vi "Lab_3_START_Clusters_Files_SUBVI_Michal_Cedro.vi"(8 "Error IN":errorcluster, 11 "HR Data Structure IN":T1 {"Raw Data"."Time" format="%<%x %.3X>T"}) -> (0 "error out":errorcluster, 3 "HR Data Structure OUT":T1 {"Raw Data"."Time" format="%<%x %.3X>T"})   [LabVIEW 2025]
uses:
  Labview-master/Lab_3/HR_Data_Structure.ctl
  Labview-master/Lab_3/Raw_Data_IN_HR.ctl
  Labview-master/Lab_3/Runner_Data_Structure.ctl
panel:
  out "HEART RATE ZONE":string[][](array[string])
  out "XY Graph":cluster{dbl[], "Heart Rate Zone":i32[]}(graph)
  out "BPM":cluster{"Time":timestamp[], "Bpm":i32[]}(graph)
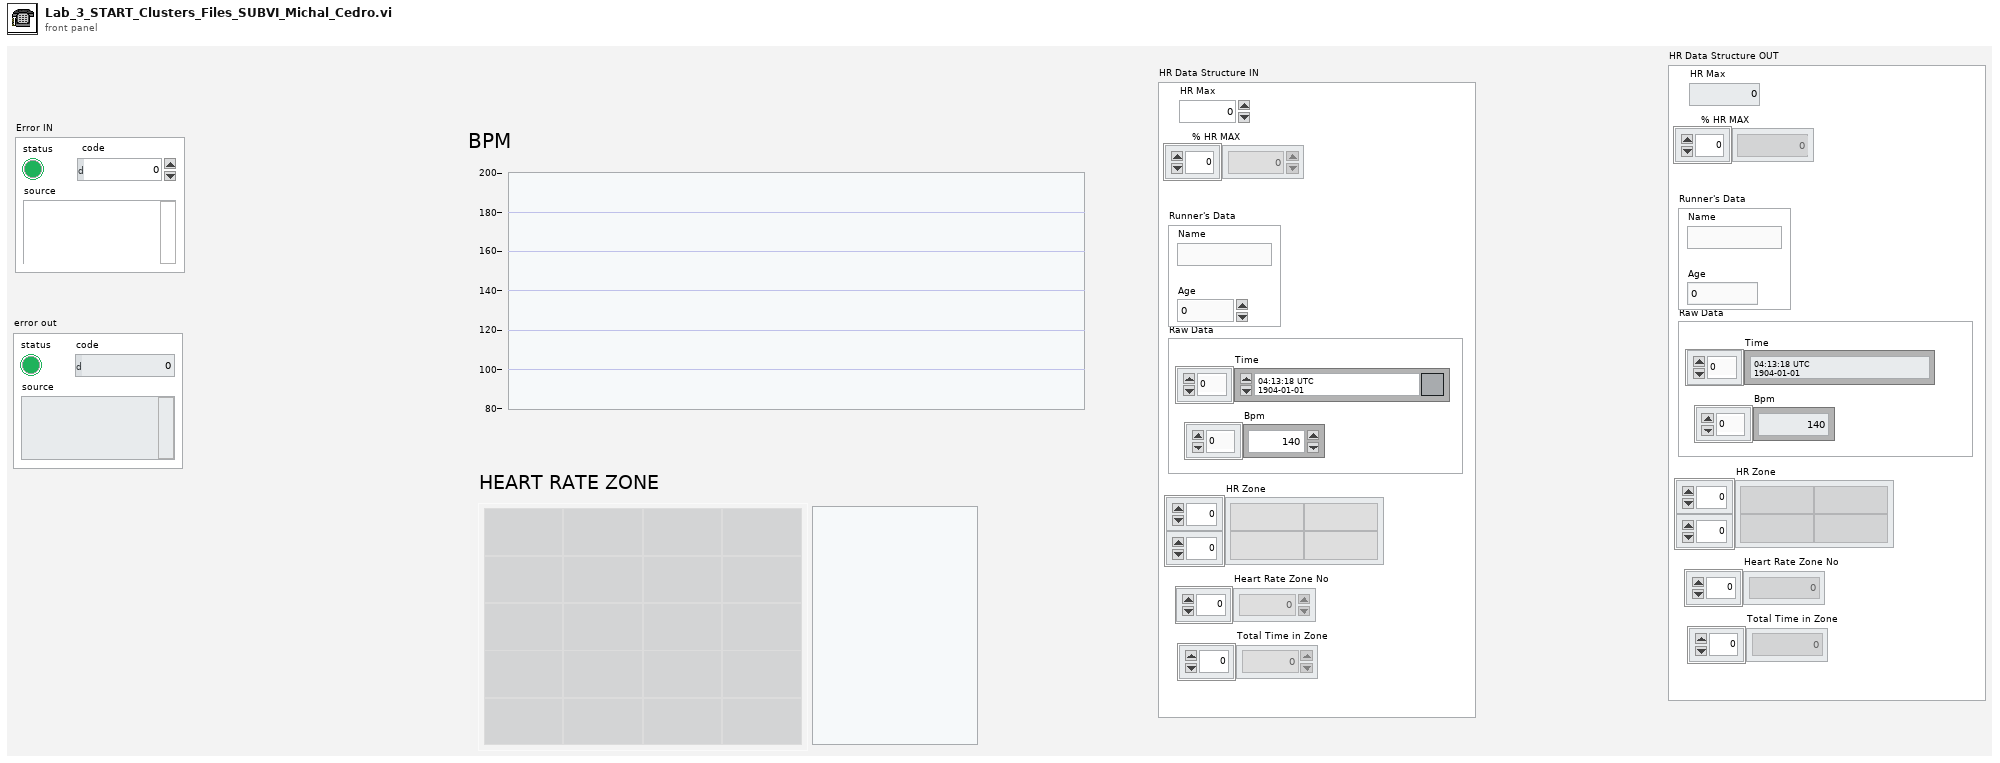
[diagram p1: front panel]
types:
  T1 = typedef "HR_Data_Structure.ctl" = cluster{"HR Max":i32, "% HR MAX ":dbl[], "Raw Data":T2, "Runner's Data":T3, "HR Zone":string[][], "Total Time in Zone":dbl[], "Heart Rate Zone No":dbl[]}
  T2 = typedef "Raw_Data_IN_HR.ctl" = cluster{"Time":timestamp[], "Bpm":i32[]}
  T3 = typedef "Runner_Data_Structure.ctl" = cluster{"Name":string, "Age":i32}
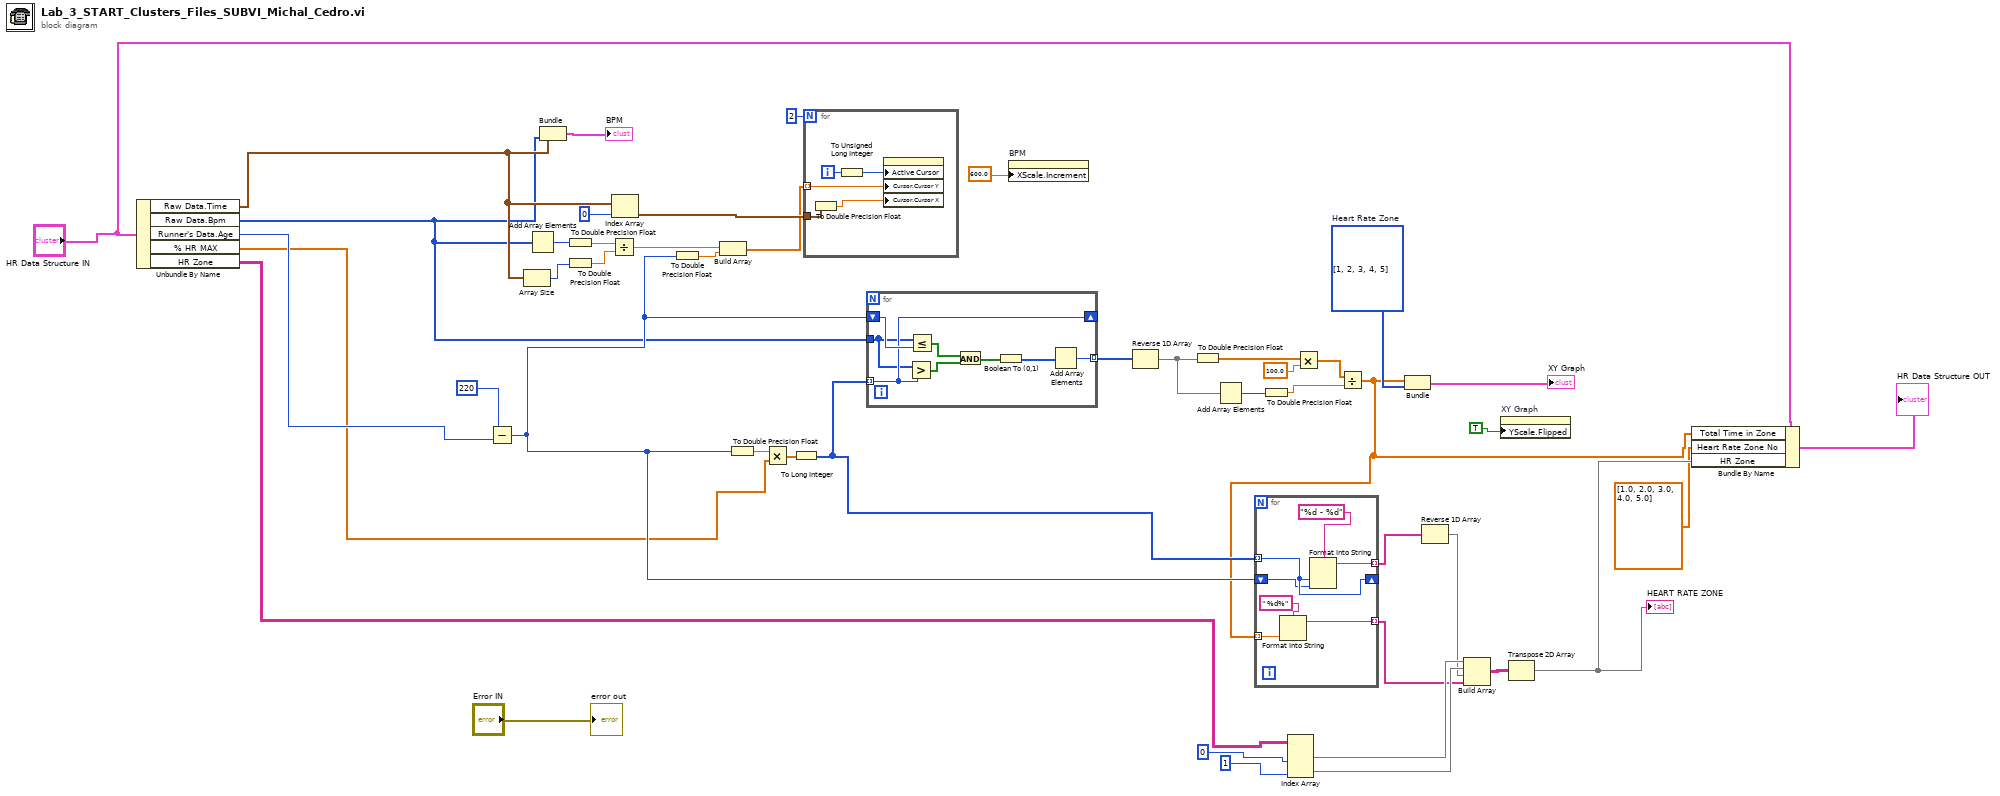
[diagram p0: block diagram]
diagram:
  w28 = i32[] [1, 2, 3, 4, 5]  # Heart Rate Zone
  n1 = Unbundle By Name("HR Data Structure IN") -> ("Raw Data.Time"=w12:timestamp[], "Raw Data.Bpm"=w11:i32[], "Runner's Data.Age"=w10:i32, "% HR MAX"=w3:dbl[], "HR Zone"=w9:string[][])
  n2 = Subtract(x=220, y=w10) -> (x-y=w25:i32)
  n3 = Array Size(array=w12) -> (size(s)=w44:i32)
  n4 = Add Array Elements(numeric array=w11) -> (sum=w45:i32)
  n5 = Bundle("Time"=w12, "Bpm"=w11) -> (→"BPM":cluster{"Time":timestamp[], "Bpm":i32[]})  [unwired: 1 in]
  n6 = To Double Precision Float(number=w45) -> (double precision float=w43:dbl)
  n7 = To Double Precision Float(number=w44) -> (double precision float=w42:dbl)
  n8 = Divide(x=w43, y=w42) -> (x/y=w26:dbl)
  n9 = Index Array(array=w12, index=0) -> (element=w38:timestamp)
  n10 = To Double Precision Float(number=w25) -> (double precision float=w5:dbl)
  n11 = Build Array(w26, w5) -> (w24:dbl[])
  n12 = To Double Precision Float(number=w25) -> (double precision float=w41:dbl)
  n13 = Multiply(x=w41, y=w3) -> (x*y=w37:dbl[])
  n14 = To Long Integer(number=w37) -> (32bit integer=w36:i32[])
  n15 = for {
    N: 2 -> [_]
    tunnel: w24 -> [w49] mode=indexing
    tunnel: w38 -> [w51]
    i -> [w48]
    n16 = To Double Precision Float(number=w51) -> (double precision float=w50:dbl)
    n17 = To Unsigned Long Integer(number=w48) -> (unsigned 32bit integer=w47:u32)
    n18 = property on="BPM" class="XYGraph (strict)"("Active Cursor"=w47, "Cursor.Cursor Y"=w49, "Cursor.Cursor X"=w50) -> ()  [unwired: 2 in, 2 out]
  }
  n19 = for {
    tunnel: w36 -> [w58] mode=indexing
    tunnel: w11 -> [w57]
    shift-right: [w58] -> _
    shift-left: w25 -> [w59]
    tunnel: [w56] -> w35 mode=indexing
    n20 = Greater?(x=w57, y=w58) -> (0:w53:bool[])
    n21 = Less Or Equal?(x=w57, y=w59) -> (x <= y?=w54:bool[])
    n22 = And(x=w54, y=w53) -> (x .and. y?=w52:bool[])
    n23 = Boolean To (0,1)(Boolean=w52) -> (0, 1=w55:i16[])
    n24 = Add Array Elements(numeric array=w55) -> (sum=w56:i16)
  }
  n25 = property on="BPM" class="XYGraph (strict)"("XScale.Increment"=600.0) -> ()  [unwired: 2 in, 2 out]
  n26 = Reverse 1D Array(array=w35) -> (reversed array=w34:i16[])
  n27 = To Double Precision Float(number=w34) -> (double precision float=w33:dbl[])
  n28 = Add Array Elements(numeric array=w34) -> (sum=w31:i16)
  n29 = To Double Precision Float(number=w31) -> (double precision float=w29:dbl)
  n30 = Index Array(array=w9, index (col) #1=0, index (col) #2=1) -> (element #1=w21:string[], element #2=w20:string[])  [unwired: 2 in]
  n31 = Multiply(x=w33, y=100.0) -> (x*y=w30:dbl[])
  n32 = Divide(x=w30, y=w29) -> (x/y=w2:dbl[])
  n33 = for {
    tunnel: w36 -> [w65] mode=indexing
    tunnel: [w66] -> w27 mode=indexing
    shift-right: [w65] -> _
    shift-left: w25 -> [w64]
    tunnel: w2 -> [w63] mode=indexing
    tunnel: [w62] -> w18 mode=indexing
    n34 = Format Into String(format string=" %d%", w63) -> (resulting string=w62:string)  [unwired: 2 in, 1 out]
    n35 = Format Into String(format string="%d - %d", w65, w64) -> (resulting string=w66:string)  [unwired: 2 in, 1 out]
  }
  n36 = Bundle(w2, "Heart Rate Zone"=w28) -> (→"XY Graph":cluster{dbl[], "Heart Rate Zone":i32[]})  [unwired: 1 in]
  n37 = Reverse 1D Array(array=w27) -> (reversed array=w19:string[])
  n38 = Build Array(w21, w20, w19, w18) -> (w17:string[][])
  n39 = property on="XY Graph" class="XYGraph (strict)"("YScale.Flipped"=TRUE) -> ()  [unwired: 2 in, 2 out]
  n40 = Transpose 2D Array(2D array=w17) -> (transposed array=w6:string[][])
  "HEART RATE ZONE" <- w6
  n41 = Bundle By Name(cluster="HR Data Structure IN", "Total Time in Zone"=w2, "Heart Rate Zone No"=dbl[] [1.0, 2.0, 3.0, 4.0, 5.0], "HR Zone"=w6) -> (→"HR Data Structure OUT":T1)
  "error out" <- "Error IN"
